vi "Draw East Wall.vi"(4 "pen":T1={"Width"=2, "Style"=enum."Solid"}, 6 "color":u32(colorbox)=11841024, 7 "Grid Size (10)":i32=10, 8 "Connected":bool, 9 "Col":i32, 10 "Row":i32, 11 "Picture In":picture) -> (3 "Picture":picture)   [LabVIEW 2020, in "App.lvlib" / "MazeUI.lvclass"]
uses:
  MazeUI.lvclass
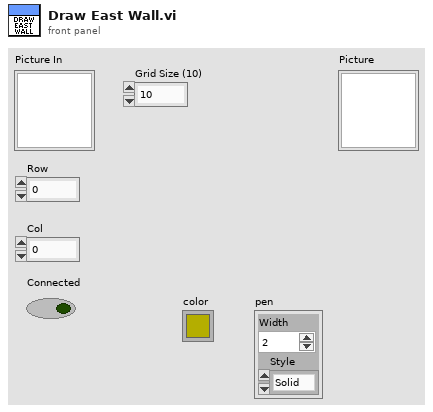
[diagram p1: front panel]
types:
  T1 = cluster{"Width":u16, "Style":enum32{"Solid", "Dash", "Dot", "DashDot", "DashDotDot"}}
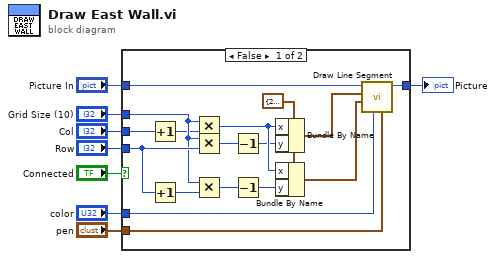
[diagram p0: block diagram]
diagram:
  n1 = case shown="False" "Connected" {
    tunnel: "Picture In" -> [w21 w26]
    tunnel: "Grid Size (10)" -> [w23 _]
    tunnel: "Row" -> [w24 _]
    tunnel: "Col" -> [w25 _]
    tunnel: "color" -> [w16 _]
    tunnel: "pen" -> [w15 _]
    tunnel: [w14 w26] -> w1
    frame False {
      w19 = cluster{"x":i16, "y":i16} {"x"=20, "y"=10} ("Start")
      n2 = Increment(x=w25) -> (x+1=w13:i32)
      n3 = Increment(x=w24) -> (x+1=w22:i32)
      n4 = Multiply(x=w23, y=w13) -> (x*y=w17:i32)
      n5 = Multiply(x=w23, y=w24) -> (x*y=w11:i32)
      n6 = Multiply(x=w23, y=w22) -> (x*y=w12:i32)
      n7 = Decrement(x=w11) -> (x-1=w10:i32)
      n8 = Decrement(x=w12) -> (x-1=w9:i32)
      n9 = Bundle By Name(cluster=w19, "x"=w17, "y"=w10) -> (w20:cluster{"x":i16, "y":i16})
      n10 = Bundle By Name(cluster=w19, "x"=w17, "y"=w9) -> (w18:cluster{"x":i16, "y":i16})
      n11 = call "Draw Line Segment.vi"("pen"=w15, "color"=w16, "End"=w18, "Start"=w20, "Picture In (New)"=w21) -> ("Picture"=w14:picture)  [unwired: 6 in]
    }
    frame True {
    }
  }
  "Picture" <- w1
